vi "GetReferences.vi"(0 "reference in":refnum<class "G#BaseAggregator.lvclass">, 5 "error in (no error)":errorcluster) -> (14 "reference out":refnum<class "G#BaseAggregator.lvclass">, 15 "G#BaseClass1.lvclass":refnum<class "G#BaseClass1.lvclass">, 16 "G#BaseClass2.lvclass":refnum<class "G#BaseClass2.lvclass">, 19 "error out":errorcluster)   [LabVIEW 2017, in "G#BaseAggregator.lvclass"]
uses:
  G#BaseAggregator.lvclass
  G#BaseClass1_class/G#BaseClass1.lvclass
  G#BaseClass2_class/G#BaseClass2.lvclass
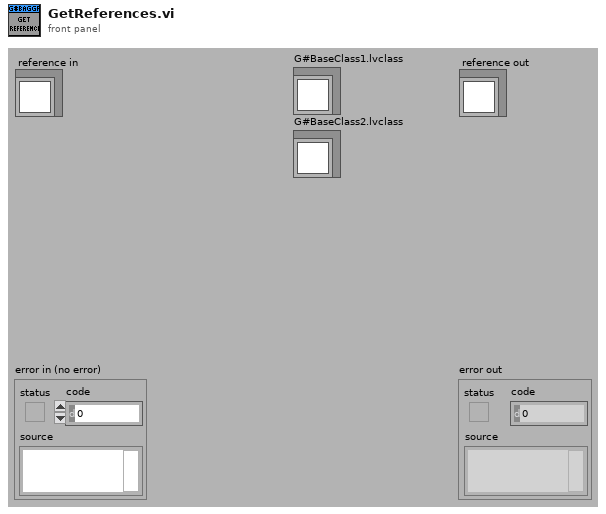
[diagram p1: front panel]
types:
  T1 = typedef "G#BaseAggregator.lvclass/ObjectAttributes.ctl" = cluster{"Numeric":dbl, "G#BaseClass1.lvclass":refnum<class "G#BaseClass1.lvclass">, "G#BaseClass2.lvclass":refnum<class "G#BaseClass2.lvclass">}
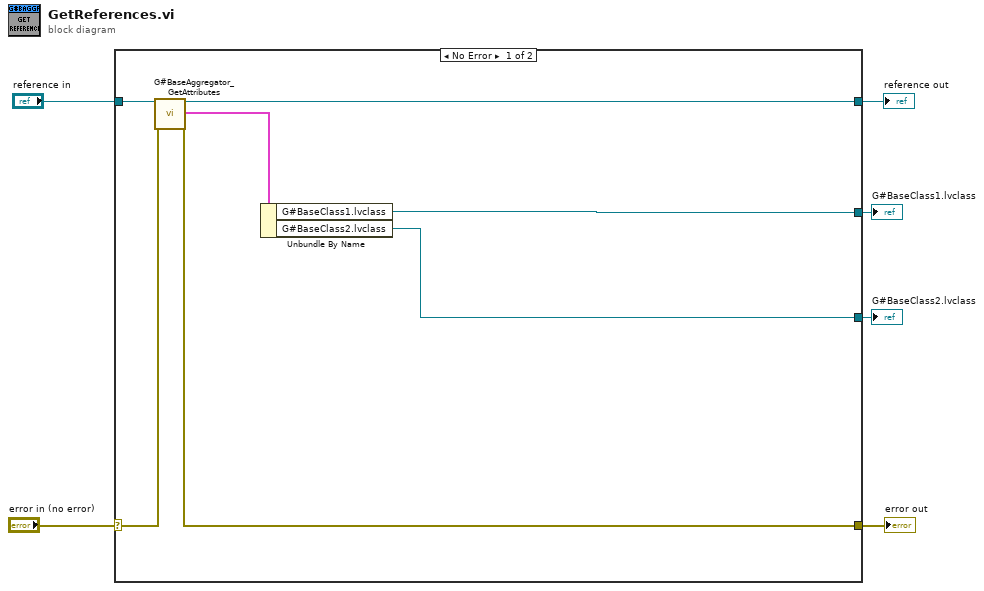
[diagram p0: block diagram]
diagram:
  n1 = case shown="No Error" "error in (no error)" {
    selector: "error in (no error)" -> [w13 w15]
    tunnel: [w12 w15] -> w5
    tunnel: [w11 w14] -> w3
    tunnel: "reference in" -> [w9 w14]
    tunnel: [w8 _] -> w2
    tunnel: [w7 _] -> w1
    frame No Error {
      n2 = call "G#BaseAggregator_GetAttributes.vi"("reference in"=w9, "error in (no error)"=w13) -> ("reference out"=w11:refnum<class "G#BaseAggregator.lvclass">, "attributes"=w10:T1, "error out"=w12:errorcluster)  [unwired: 14 in, 1 out]
      n3 = Unbundle By Name(w10) -> ("G#BaseClass1.lvclass"=w8:refnum<class "G#BaseClass1.lvclass">, "G#BaseClass2.lvclass"=w7:refnum<class "G#BaseClass2.lvclass">)
    }
    frame Error {
    }
  }
  "error out" <- w5
  "reference out" <- w3
  "G#BaseClass1.lvclass" <- w2
  "G#BaseClass2.lvclass" <- w1
